vi "FlatToRichni_protobuf_types_PrecisionTimestamp.vi"(5 "OutputClusterType":T1, 11 "InputCluster":T2) -> (3 "OutputCluster":T1)   [LabVIEW 2021, in "ni.protobuf.types.lvlib"]
uses:
  ni.protobuf.types.lvlib
  ni_protobuf_types_PrecisionTimestamp_Flat.ctl
  ni_protobuf_types_PrecisionTimestamp.ctl
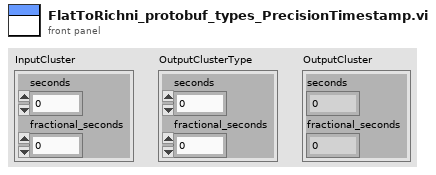
[diagram p1: front panel]
types:
  T1 = typedef "ni.protobuf.types.lvlib/ni_protobuf_types_PrecisionTimestamp.ctl" = cluster{"seconds":i64, "fractional_seconds":u64}
  T2 = typedef "ni.protobuf.types.lvlib/ni_protobuf_types_PrecisionTimestamp_Flat.ctl" = cluster{"seconds":i64, "fractional_seconds":u64}
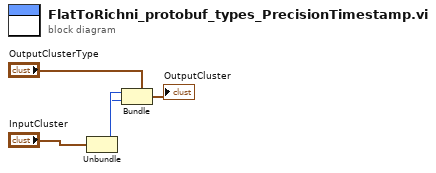
[diagram p0: block diagram]
diagram:
  n1 = Unbundle "Unbundle"("InputCluster") -> ("seconds"=w2:i64, "fractional_seconds"=w1:u64)
  n2 = Bundle "Bundle"(cluster="OutputClusterType", "seconds"=w2, "fractional_seconds"=w1) -> (→"OutputCluster":T1)
